vi "Tank_Feedback.vi"() -> (3 "Comment":string)   [LabVIEW 2010]
uses:
  ADAM Client/Sub VIs/ADAM Controls/Address.ctl
panel:
  out "Salt Saturator Level":dbl format="%.3f"
  out "Tank D Level":dbl format="%.3f"
  out "Tank C Level":dbl format="%.3f"
  out "Tank B Level":dbl format="%.3f"
  out "Tank A Level":dbl format="%.3f"
  out "Sub2":cluster{"State":bool, "name":string}[](array[cluster])
  out "Sub1":cluster{"State":bool, "name":string}[](array[cluster])
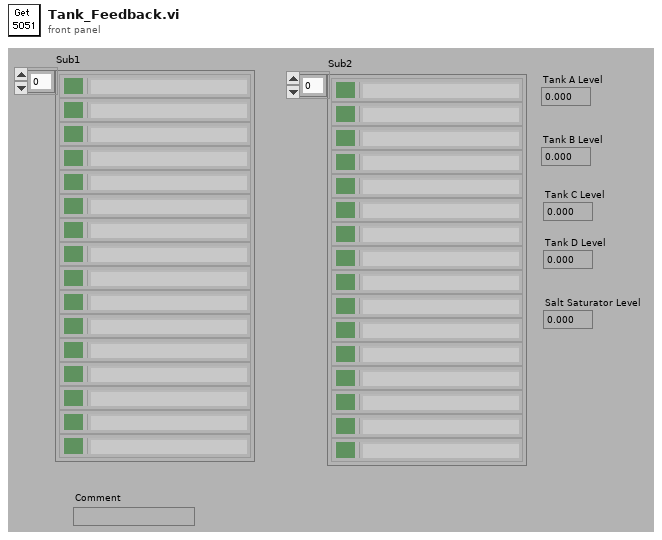
[diagram p1: front panel]
types:
  T1 = typedef "Address.ctl" = cluster{"Main":i32, "Ch.":i32, "Sub":i32, "Port Name":string}
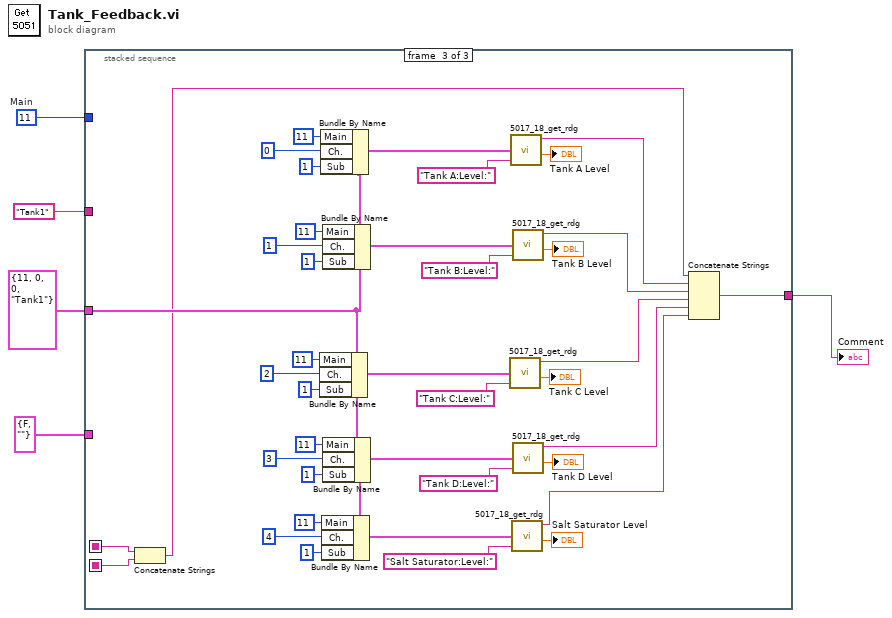
[diagram p0: block diagram]
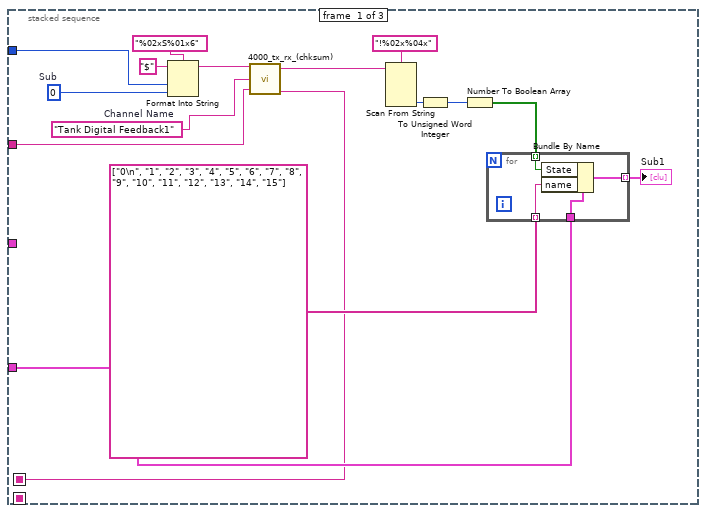
[diagram p2: hidden frame]
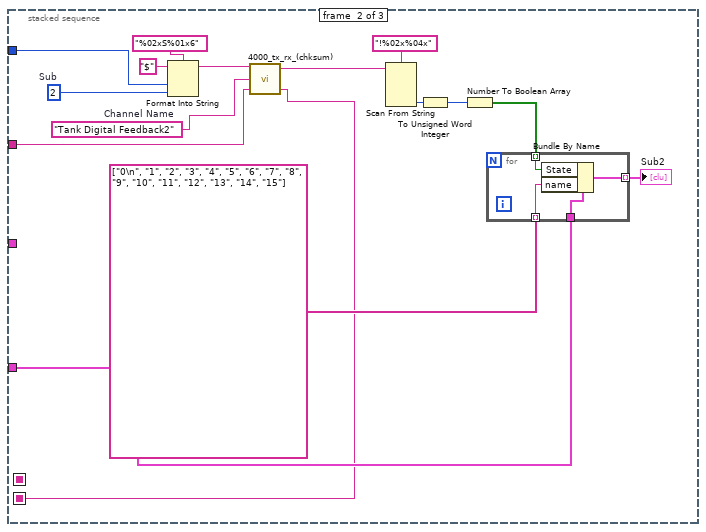
[diagram p3: hidden frame]
diagram:
  w4 = 11  # Main
  n1 = stacked-sequence {
    seq-local: [_ w26 _] -> [_ _ w53]
    seq-local: [w6 _ _] -> [_ _ w54]
    tunnel: "Tank1" ("Port Name") -> [w14 w34 _]
    tunnel: w4 -> [w13 w33 _]
    tunnel: cluster{"State":bool, "name":string} {"State"=FALSE, "name"=""} ("Cluster") -> [w10 w30 _]
    tunnel: T1 {"Main"=11, "Ch."=0, "Sub"=0, "Port Name"="Tank1"} ("Address (all reqd.)") -> [_ _ w55]
    tunnel: [_ _ w46] -> w1
    frame #0 {
      w11 = "Tank Digital Feedback1"  # Channel Name
      w12 = 0  # Sub
      n2 = Format Into String(format string="%02xS%01x6", initial string="$", w13, w12) -> (resulting string=w19:string)  [unwired: 1 in, 1 out]
      n3 = call "4000_tx_rx_(chksum).vi"("Port Name"=w14, "Channel Name"=w11, "Write String"=w19) -> ("Comment out"=w6:string, "Read"=w18:string)  [unwired: 1 out]
      n4 = Scan From String(format string="!%02x%04x", input string=w18) -> (output 2=w15:i32)  [unwired: 2 in, 6 out]
      n5 = To Unsigned Word Integer(number=w15) -> (unsigned 16bit integer=w17:u16)
      n6 = Number To Boolean Array(number=w17) -> (Boolean array=w9:bool[])
      n7 = for {
        tunnel: w10 -> [w25]
        tunnel: w9 -> [w24] mode=indexing
        tunnel: string[] ["0\n", "1", "2", "3", "4", "5", "6", "7", "8", "9", "10", "11", "12", "13", "14", "15"] -> [w23] mode=indexing
        tunnel: [w22] -> w7 mode=indexing
        n8 = Bundle By Name(cluster=w25, "State"=w24, "name"=w23) -> (w22:cluster{"State":bool, "name":string})
      }
      "Sub1" <- w7
    }
    frame #1 {
      w31 = "Tank Digital Feedback2"  # Channel Name
      w32 = 2  # Sub
      n9 = Format Into String(format string="%02xS%01x6", initial string="$", w33, w32) -> (resulting string=w39:string)  [unwired: 1 in, 1 out]
      n10 = call "4000_tx_rx_(chksum).vi"("Port Name"=w34, "Channel Name"=w31, "Write String"=w39) -> ("Comment out"=w26:string, "Read"=w38:string)  [unwired: 1 out]
      n11 = Scan From String(format string="!%02x%04x", input string=w38) -> (output 2=w35:i32)  [unwired: 2 in, 6 out]
      n12 = To Unsigned Word Integer(number=w35) -> (unsigned 16bit integer=w37:u16)
      n13 = Number To Boolean Array(number=w37) -> (Boolean array=w29:bool[])
      n14 = for {
        tunnel: w30 -> [w45]
        tunnel: w29 -> [w44] mode=indexing
        tunnel: string[] ["0\n", "1", "2", "3", "4", "5", "6", "7", "8", "9", "10", "11", "12", "13", "14", "15"] -> [w43] mode=indexing
        tunnel: [w42] -> w27 mode=indexing
        n15 = Bundle By Name(cluster=w45, "State"=w44, "name"=w43) -> (w42:cluster{"State":bool, "name":string})
      }
      "Sub2" <- w27
    }
    frame #2 {
      n16 = Concatenate Strings(w54, w53) -> (w52:string)
      n17 = Bundle By Name(cluster=w55, "Main"=11, "Ch."=2, "Sub"=1) -> (w70:T1)
      n18 = Bundle By Name(cluster=w55, "Main"=11, "Ch."=0, "Sub"=1) -> (w82:T1)
      n19 = Bundle By Name(cluster=w55, "Main"=11, "Ch."=4, "Sub"=1) -> (w58:T1)
      n20 = Bundle By Name(cluster=w55, "Main"=11, "Ch."=1, "Sub"=1) -> (w77:T1)
      n21 = Bundle By Name(cluster=w55, "Main"=11, "Ch."=3, "Sub"=1) -> (w65:T1)
      n22 = call "5017_18_get_rdg.vi"("Address (all reqd.)"=w70, "Channel Name"="Tank C:Level:") -> ("Comment"=w49:string, "Reading"=→"Tank C Level":dbl)  [unwired: 3 in]
      n23 = call "5017_18_get_rdg.vi"("Address (all reqd.)"=w82, "Channel Name"="Tank A:Level:") -> ("Comment"=w51:string, "Reading"=→"Tank A Level":dbl)  [unwired: 3 in]
      n24 = call "5017_18_get_rdg.vi"("Address (all reqd.)"=w58, "Channel Name"="Salt Saturator:Level:") -> ("Comment"=w47:string, "Reading"=→"Salt Saturator Level":dbl)  [unwired: 3 in]
      n25 = call "5017_18_get_rdg.vi"("Address (all reqd.)"=w77, "Channel Name"="Tank B:Level:") -> ("Comment"=w50:string, "Reading"=→"Tank B Level":dbl)  [unwired: 3 in]
      n26 = call "5017_18_get_rdg.vi"("Address (all reqd.)"=w65, "Channel Name"="Tank D:Level:") -> ("Comment"=w48:string, "Reading"=→"Tank D Level":dbl)  [unwired: 3 in]
      n27 = Concatenate Strings(w52, w51, w50, w49, w48, w47) -> (w46:string)
    }
  }
  "Comment" <- w1
